vi "fgv_calib_(refer).vi"(7 "State":enum16{"Write", "Read"}(ring), 8 "error in (no error)":errorcluster, 9 "enclosure box IN":T1 {"Rotation" format="%.2f"; "Left" scale=0.0..1024.0; "Right" scale=0.0..1024.0}, 10 "Location in Pixels":T3(array[cluster]), 11 "Reference Image":T2 caption="Original Image") -> (0 "error in (no error)":errorcluster, 1 "enclosure box OUT":T1 {"Rotation" format="%.2f"; "Left" scale=0.0..1024.0; "Right" scale=0.0..1024.0}, 2 "Location in Pixels":T3(array[cluster]), 3 "Reference Image":T2 caption="Original Image")   [LabVIEW 2020]
uses:
  <vilib>/vision/Image Controls.llb/IMAQ Image.ctl
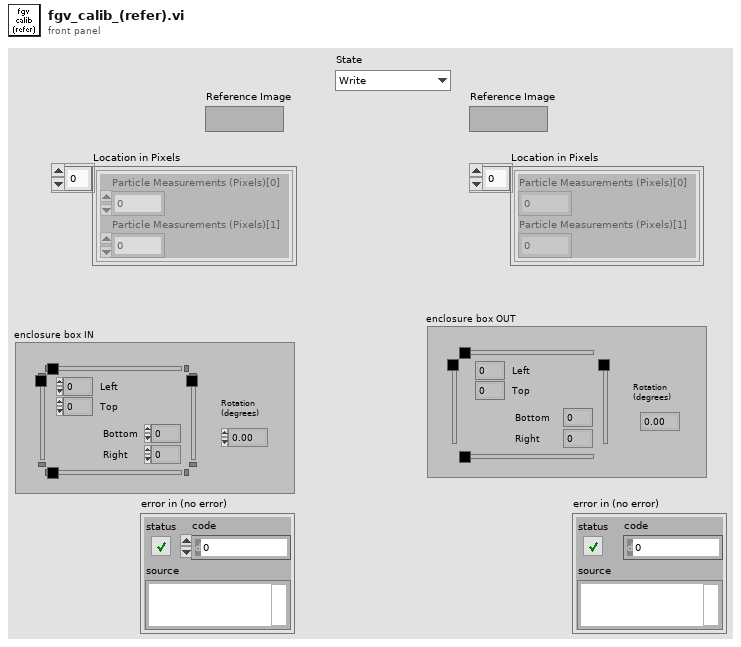
[diagram p1: front panel]
types:
  T1 = typedef "IMAQ Rectangle" = cluster{"Left":i32, "Top":i32, "Right":i32, "Bottom":i32, "Rotation":dbl}
  T2 = typedef "IMAQ Image.ctl" = refnum<image>
  T3 = cluster{"Particle Measurements (Pixels)[0]":dbl, "Particle Measurements (Pixels)[1]":dbl}[]
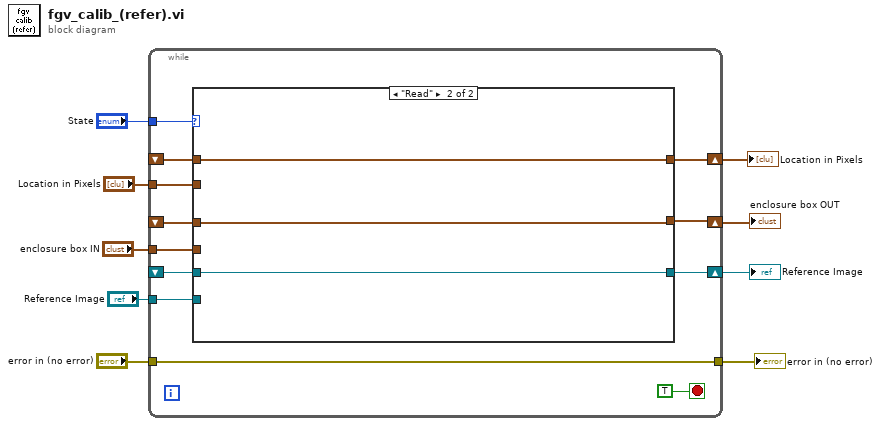
[diagram p0: block diagram]
diagram:
  n1 = while {
    tunnel: "State" -> [w20]
    tunnel: "Location in Pixels" -> [w19]
    shift-right: [w18] -> w7
    shift-left: _ -> [w17]
    tunnel: "Reference Image" -> [w16]
    shift-right: [w15] -> w5
    shift-left: _ -> [w14]
    tunnel: "error in (no error)" -> [w13]
    tunnel: [w13] -> w3
    shift-right: [w11] -> w1
    shift-left: _ -> [w12]
    tunnel: "enclosure box IN" -> [w10]
    stop <- TRUE stop-if-true
    n2 = case shown="\"Read\"" w20 {
      tunnel: w19 -> [w24 _]
      tunnel: [w24 w27] -> w18
      tunnel: w17 -> [_ w27]
      tunnel: w16 -> [w23 _]
      tunnel: [w23 w26] -> w15
      tunnel: w14 -> [_ w26]
      tunnel: [w22 w25] -> w11
      tunnel: w12 -> [_ w25]
      tunnel: w10 -> [w22 _]
      frame "Write", Default {
      }
      frame "Read" {
      }
    }
  }
  "error in (no error)" <- w3
  "Location in Pixels" <- w7
  "Reference Image" <- w5
  "enclosure box OUT" <- w1
